vi "TRStimestampCheck.vi"(10 "element":u32 format="%032b") -> (2 "TRSTimestamp?":bool)   [LabVIEW 2014]
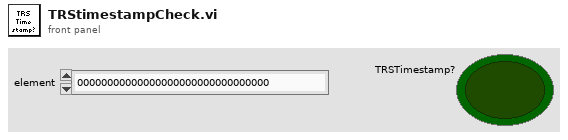
[diagram p1: front panel]
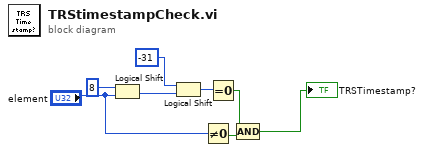
[diagram p0: block diagram]
diagram:
  n1 = Logical Shift(y=i16 8, x="element") -> (x << y=w6:u32)
  n2 = Logical Shift(y=i16 -31, x=w6) -> (x << y=w5:u32)
  n3 = Not Equal To 0?(x="element") -> (x != 0?=w1:bool)
  n4 = Equal To 0?(x=w5) -> (x = 0?=w4:bool)
  n5 = Compound Arithmetic op=AND(w4, w1) -> (→"TRSTimestamp?":bool)
